vi "2photocell.vi"() -> ()   [LabVIEW 2016]
uses:
  <vilib>/LabVIEW Interface for Arduino/LabVIEW Interface for Arduino.lvlib
  <vilib>/ptbypt/NI_PtbyPt.lvlib
panel:
  out "Filtered x 2":dbl format="%0.2f"
  out "Filtered x":dbl format="%0.2f"
  in  "Duty Cycle (0 - 255)":u8
  out "Light Intensity\nPhotosell 2\n(0 - 100) 2":dbl(knob) scale=0.0..100.0
  out "Light Intensity \nPhotocell 1\n(0 - 100)":dbl(knob) scale=0.0..100.0
  in  "stop":bool
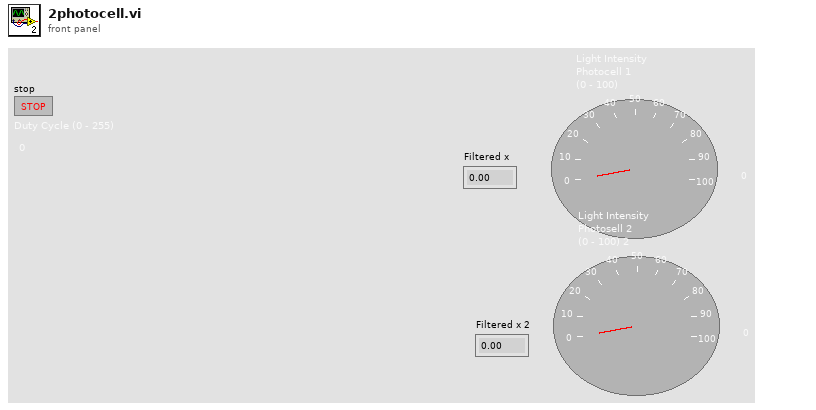
[diagram p1: front panel]
types:
  T1 = typedef "LabVIEW Interface for Arduino.lvlib/Arduino Resource.ctl" = cluster{"VISA resource":refnum<visa-resource-name>, "Board Type":T2, "Connection Type":enum8{"USB / Serial"}, "Bytes Per Packet (15)":u8}
  T2 = typedef "LabVIEW Interface for Arduino.lvlib/Board Type.ctl" = enum16{"Uno", "Dimuelanove w/Atmega 328", "Mega 2560"}
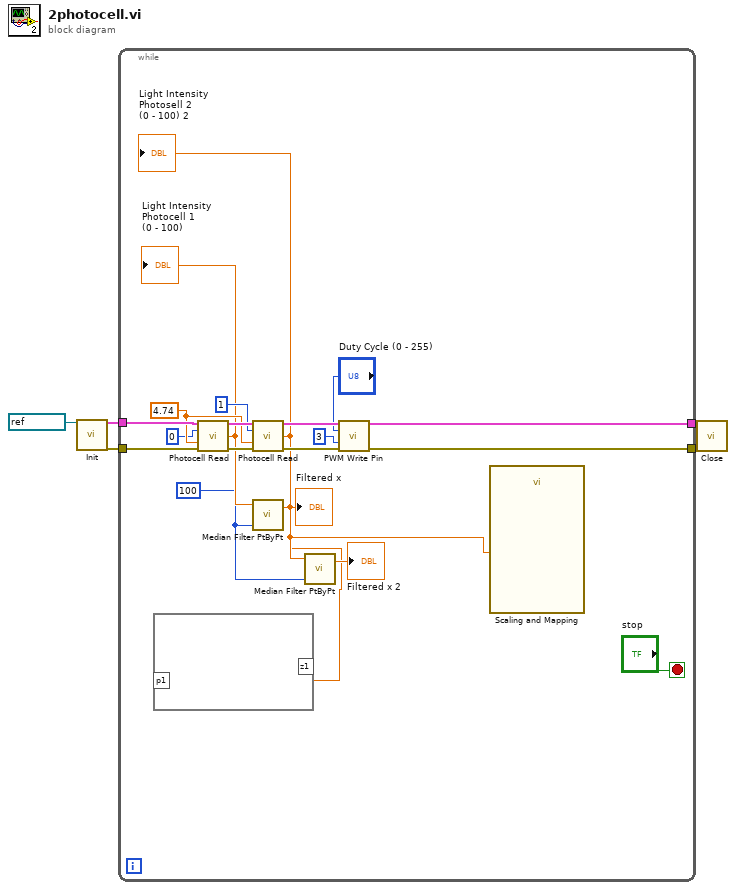
[diagram p0: block diagram]
diagram:
  n1 = call <vilib>:"Init.vi"("VISA resource"=refnum<visa-resource-name> "COM3") -> ("Arduino Resource"=w4:T1, "error out"=w2:errorcluster)  [unwired: 17 in]
  n2 = while {
    tunnel: w4 -> [w23]
    tunnel: [w20] -> w3
    tunnel: w2 -> [w19]
    tunnel: [w16] -> w1
    stop <- "stop" stop-if-true
    w7 = 100
    w15 = 4.74
    n3 = call <vilib>:"Photocell Read.vi"("Arduino Resource"=w23, "Photo Cell Pin (0)"=u8 0, "Vcc (5)"=w15, "error in"=w19) -> ("Arduino Resource"=w22:T1, "Light Intensity (0 - 100)"=w10:dbl, "error out"=w18:errorcluster)  [unwired: 9 in]
    "Light Intensity \nPhotocell 1\n(0 - 100)" <- w10
    n4 = call <vilib>:"Photocell Read.vi"("Arduino Resource"=w22, "Photo Cell Pin (0)"=u8 1, "Vcc (5)"=w15, "error in"=w18) -> ("Arduino Resource"=w21:T1, "Light Intensity (0 - 100)"=w8:dbl, "error out"=w17:errorcluster)  [unwired: 9 in]
    "Light Intensity\nPhotosell 2\n(0 - 100) 2" <- w8
    n5 = call <vilib>:"Median Filter PtByPt.vi"("rank"=w7, "x"=w10) -> ("Filtered x"=w6:dbl)  [unwired: 2 in, 1 out]
    "Filtered x" <- w6
    n6 = formula code=""("p1"=w6) -> ()  [unwired: 1 out]
    n7 = call <vilib>:"Median Filter PtByPt.vi"("rank"=w7, "x"=w8) -> ("Filtered x"=→"Filtered x 2":dbl)  [unwired: 2 in, 1 out]
    n8 = call <vilib>:"PWM Write Pin.vi"("Arduino Resource"=w21, "Duty Cycle (0 - 255)"="Duty Cycle (0 - 255)", "PWM Pin (3)"=u8 3, "error in"=w17) -> ("Arduino Resource"=w20:T1, "error out"=w16:errorcluster)  [unwired: 10 in]
    n9 = call "Scaling and Mapping"("Signals"=w6) -> ()  [unwired: 9 in, 2 out]
  }
  n10 = call <vilib>:"Close.vi"("Arduino Resource"=w3, "error in"=w1) -> ()  [unwired: 13 in, 1 out]
